vi "Initialize.vi"(8 "error in (no error)":errorcluster, 11 "RS232 in":refnum<class "RS-xxx.lvclass">) -> (0 "error out":errorcluster, 3 "RS232 out":refnum<class "RS-xxx.lvclass">)   [LabVIEW 2023, in "Protocols.lvlib" / "RS-xxx.lvclass"]
uses:
  RS-xxx.lvclass
  <vilib>/Instr/_visa.llb/VISA Configure Serial Port (Instr).vi
  Protocol Parent/Protocol Parent.lvclass
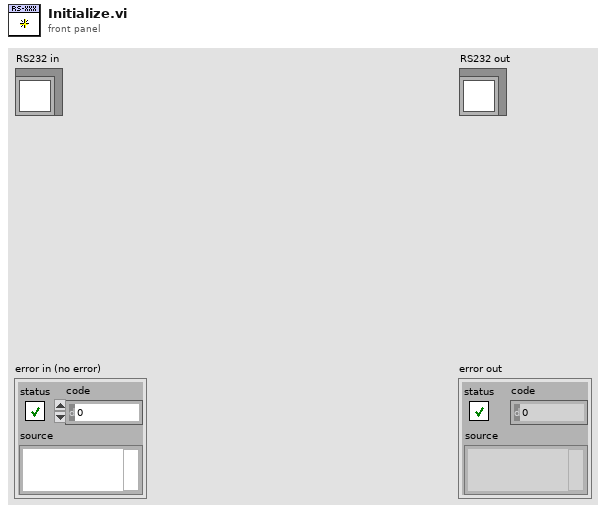
[diagram p1: front panel]
types:
  T1 = cluster{"Port":string, "Baud Rate":u32, "Data Bits":u16, "Parity":enum16{"None", "Odd", "Even", "Mark", "Space"}, "Stop Bits":u16, "Flow Control":u16, "XON":enum16{"NUL", "SOH", "STX", "ETX", "EOT", "ENQ", "ACK", "BEL", "BS", "HT", "LF", "VT", "FF", "CR", "SO", "SI", "DLE", "DC1", "DC2", "DC3", "DC4", "NAK", "SYN", "ETB", "CAN", "EM", "SUB", "ESC", "FS", "GS", "RS", "US", "SP", "!", "\"", "#", "$", "%", "&", "'", "(", ")", "*", "+", ",", "- (-)", ".", "/", "0", "1", "2", "3", "4", "5", "6", "7", "8", "9", ":", ";", "<", "=", ">", "?", "@", "A", "B", "C", "D", "E", "F", "G", "H", "I", "J", "K", "L", "M", "N", "O", "P", "Q", "R", "S", "T", "U", "V", "W", "X", "Y", "Z", "[", "\\", "]", "^", "_", "`", "a", "b", "c", "d", "e", "f", "g", "h", "i", "j", "k", "l", "m", "n", "o", "p", "q", "r", "s", "t", "u", "v", "w", "x", "y", "z", "{", "|", "}", "~"}, "XOFF":enum16{"NUL", "SOH", "STX", "ETX", "EOT", "ENQ", "ACK", "BEL", "BS", "HT", "LF", "VT", "FF", "CR", "SO", "SI", "DLE", "DC1", "DC2", "DC3", "DC4", "NAK", "SYN", "ETB", "CAN", "EM", "SUB", "ESC", "FS", "GS", "RS", "US", "SP", "!", "\"", "#", "$", "%", "&", "'", "(", ")", "*", "+", ",", "- (-)", ".", "/", "0", "1", "2", "3", "4", "5", "6", "7", "8", "9", ":", ";", "<", "=", ">", "?", "@", "A", "B", "C", "D", "E", "F", "G", "H", "I", "J", "K", "L", "M", "N", "O", "P", "Q", "R", "S", "T", "U", "V", "W", "X", "Y", "Z", "[", "\\", "]", "^", "_", "`", "a", "b", "c", "d", "e", "f", "g", "h", "i", "j", "k", "l", "m", "n", "o", "p", "q", "r", "s", "t", "u", "v", "w", "x", "y", "z", "{", "|", "}", "~"}, "End Read on Termination Character":bool, "End Write on Termination Character":bool, "Termination Character":u8, "4wireMode":bool, "AssertDTR":bool, "WireMode":i16}
  T2 = enum16{"NUL", "SOH", "STX", "ETX", "EOT", "ENQ", "ACK", "BEL", "BS", "HT", "LF", "VT", "FF", "CR", "SO", "SI", "DLE", "DC1", "DC2", "DC3", "DC4", "NAK", "SYN", "ETB", "CAN", "EM", "SUB", "ESC", "FS", "GS", "RS", "US", "SP", "!", "\"", "#", "$", "%", "&", "'", "(", ")", "*", "+", ",", "- (-)", ".", "/", "0", "1", "2", "3", "4", "5", "6", "7", "8", "9", ":", ";", "<", "=", ">", "?", "@", "A", "B", "C", "D", "E", "F", "G", "H", "I", "J", "K", "L", "M", "N", "O", "P", "Q", "R", "S", "T", "U", "V", "W", "X", "Y", "Z", "[", "\\", "]", "^", "_", "`", "a", "b", "c", "d", "e", "f", "g", "h", "i", "j", "k", "l", "m", "n", "o", "p", "q", "r", "s", "t", "u", "v", "w", "x", "y", "z", "{", "|", "}", "~"}
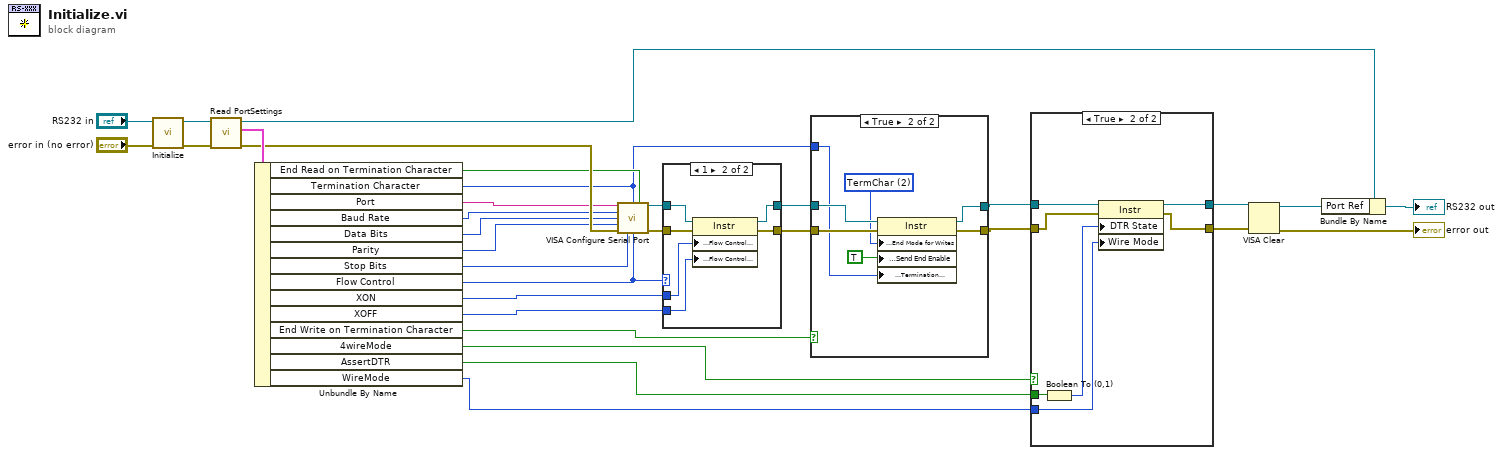
[diagram p0: block diagram]
diagram:
  n1 = call-parent "Initialize.vi"("error in (no error)"="error in (no error)", "Protocol Parent in"="RS232 in") -> ("error out"=w29:errorcluster, "Protocol Parent out"=w30:refnum<class "RS-xxx.lvclass">)  [unwired: 8 in]
  n2 = call "Read PortSettings.vi"("error in (no error)"=w29, "RS232 in"=w30) -> ("error out"=w27:errorcluster, "PortSettings"=w28:T1, "RS232 out"=w11:refnum<class "RS-xxx.lvclass">)  [unwired: 7 in]
  n3 = Unbundle By Name(w28) -> ("End Read on Termination Character"=w19:bool, "Termination Character"=w12:u8, "Port"=w26:string, "Baud Rate"=w25:u32, "Data Bits"=w24:u16, "Parity"=w23:enum16{"None", "Odd", "Even", "Mark", "Space"}, "Stop Bits"=w22:u16, "Flow Control"=w17:u16, "XON"=w18:T2, "XOFF"=w16:T2, "End Write on Termination Character"=w13:bool, "4wireMode"=w3:bool, "AssertDTR"=w2:bool, "WireMode"=w1:i16)
  n4 = call-poly "VISA Configure Serial Port"("VISA resource name"=w26, "termination char\n(0xA = '\\n' = LF)"=w12, "Enable Termination\nChar (T)"=w19, "baud rate (9600)"=w25, "data bits (8)"=w24, "parity (0:none)"=w23, "error in (no error)"=w27, "stop bits (10: 1 bit)"=w22, "flow control (0:none)"=w17) -> ("VISA resource name out"=w14:refnum<visa-resource-name>, "error out"=w15:errorcluster)  [unwired: 5 in]
  n5 = case shown="1" w17 {
    tunnel: [w33 w40] -> w20
    tunnel: [w34 w39] -> w21
    tunnel: w15 -> [w33 w38]
    tunnel: w14 -> [w34 w37]
    tunnel: w18 -> [_ w36]
    tunnel: w16 -> [_ w35]
    frame Default {
    }
    frame 1 {
      n6 = property class="Instr"(reference=w37, error in=w38, "Serial Settings:Flow Control XON Character"=w36, "Serial Settings:Flow Control XOFF Character"=w35) -> (reference out=w39:refnum<visa-resource-name>, error out=w40:errorcluster)
    }
  }
  n7 = case shown="True" w13 {
    tunnel: w21 -> [w41 w49]
    tunnel: w20 -> [w42 w48]
    tunnel: [w41 w47] -> w6
    tunnel: [w42 w46] -> w4
    tunnel: w12 -> [_ w44]
    frame False {
    }
    frame True {
      w45 = u16 2 items=["None", "LastBit", "TermChar", "Break"] ("Serial Settings:Serial End Mode for Writes")
      n8 = property class="Instr"(reference=w49, error in=w48, "Serial Settings:End Mode for Writes"=w45, "Message Based Settings:Send End Enable"=TRUE, "Message Based Settings:Termination Character"=w44) -> (reference out=w47:refnum<visa-resource-name>, error out=w46:errorcluster)
    }
  }
  n9 = case shown="True" w3 {
    tunnel: [w51 w52] -> w7
    tunnel: w6 -> [w51 w58]
    tunnel: [w50 w53] -> w5
    tunnel: w4 -> [w50 w57]
    tunnel: w2 -> [_ w56]
    tunnel: w1 -> [_ w54]
    frame False {
    }
    frame True {
      n10 = Boolean To (0,1)(Boolean=w56) -> (0, 1=w55:i16)
      n11 = property class="Instr"(reference=w58, error in=w57, "DTR State"=w55, "Wire Mode"=w54) -> (reference out=w52:refnum<visa-resource-name>, error out=w53:errorcluster)
    }
  }
  n12 = VISA Clear(VISA resource name=w7, error in (no error)=w5) -> (VISA resource name out=w9:refnum<visa-resource-name>, error out=→"error out":errorcluster)
  n13 = Bundle By Name(cluster=w11, "Port Ref"=w9) -> (→"RS232 out":refnum<class "RS-xxx.lvclass">)
